vi "UDT_loggingModule_Postrun.vi"() -> (3 "Unit Test Framework Results":T1)   [LabVIEW 2017]
doc: "Use this template to create a user-defined test VI. Define your test requirements and wire the results to the <b>Result (Test)</b> control. Do not modify the <b>Unit Test Framework Results</b> indicator."
uses:
  <vilib>/utf/common/utf_test_result_troll.ctl
  <vilib>/utf/common/utf_test_result.ctl
  <vilib>/utf/common/utf_test_result_failure.ctl
  <vilib>/utf/common/utf_test_comparison_operators.ctl
  <vilib>/utf/common/utf_vi_tag.ctl
  RT/loggingModule/Queue/TypeDefs/queueFGVState.ctl
  RT/loggingModule/Queue/TypeDefs/message.ctl
  <vilib>/Control Software Solutions Ltd/UTF Helper/SubVIs/UTF Variant Equals.vi
  <vilib>/Control Software Solutions Ltd/UTF Helper/Unit Test Helper.lvlib
  RT/loggingModule/loggingModule.lvlib
  <vilib>/utf/NI_UnitTestFramework.lvlib
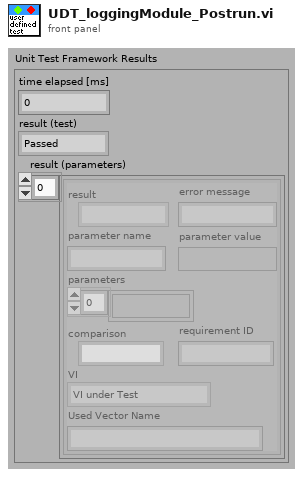
[diagram p1: front panel]
types:
  T1 = typedef "NI_UnitTestFramework.lvlib/utf_test_result_troll.ctl" = cluster{"time elapsed [ms]":u32, "result (test)":T2, "result (parameters)":T3[]}
  T2 = typedef "NI_UnitTestFramework.lvlib/utf_test_result.ctl" = enum16{"Passed", "Failed", "Error", "Skipped", "Not Processed"}
  T3 = typedef "NI_UnitTestFramework.lvlib/utf_test_result_failure.ctl" = cluster{"result":T2, "error message":string, "parameter name":string, "parameter value":variant, "parameters":variant[], "comparison":T4, "requirement ID":string, "VI":T5, "Used Vector Name":string}
  T4 = typedef "NI_UnitTestFramework.lvlib/utf_test_comparison_operators.ctl" = enum16{"=", "!=", ">", ">=", "<", "<=", "range", "symmetric tolerance", "asymmetric tolerance", "string contains", "string not contain", "array size", "string length", "array range", "by element", "array range (limit array)", "user-defined", "array contains", "array not contain", "vector length", "= (elm)", "!= (elm)", "= (case insensitive)", "!= (case insensitive)"}
  T5 = typedef "NI_UnitTestFramework.lvlib/utf_vi_tag.ctl" = enum16{"Setup VI", "VI under Test", "Teardown VI"}
  T6 = typedef "loggingModule.lvlib/message.ctl" = cluster{"calling module":string, "message":string, "data":variant}
  T7 = typedef "loggingModule.lvlib/queueFGVState.ctl" = enum16{"obtain", "enqueue low priority", "enqueue high priority", "dequeue", "release"}
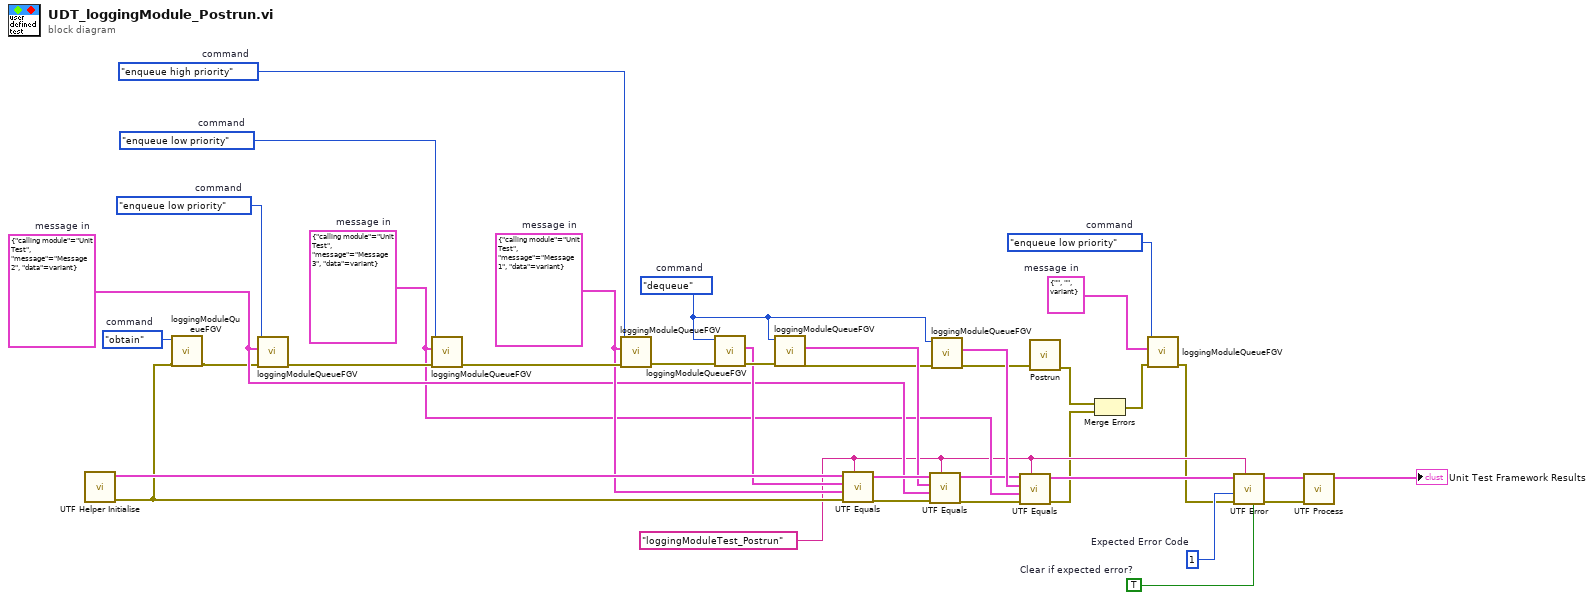
[diagram p0: block diagram]
diagram:
  w5 = TRUE  # Clear if expected error?
  w6 = 1  # Expected Error Code
  w11 = T6 {"calling module"="", "message"="", "data"=variant}  # message in
  w12 = queueFGVState."enqueue low priority"  # command
  w14 = queueFGVState."obtain"  # command
  w7 = "loggingModuleTest_Postrun"
  w22 = queueFGVState."dequeue"  # command
  w31 = T6 {"calling module"="Unit Test", "message"="Message 1", "data"=variant}  # message in
  w18 = T6 {"calling module"="Unit Test", "message"="Message 3", "data"=variant}  # message in
  w24 = T6 {"calling module"="Unit Test", "message"="Message 2", "data"=variant}  # message in
  w34 = queueFGVState."enqueue high priority"  # command
  w36 = queueFGVState."enqueue low priority"  # command
  w37 = queueFGVState."enqueue low priority"  # command
  n1 = call <vilib>:"UTF Helper Initialise.vi"() -> ("error out"=w16:errorcluster, "results array"=w32:T3[])  [unwired: 10 in]
  n2 = call "loggingModuleQueueFGV.vi"("error in (no error)"=w16, "command"=w14) -> ("error out"=w15:errorcluster)  [unwired: 8 in, 1 out]
  n3 = call "loggingModuleQueueFGV.vi"("error in (no error)"=w15, "message in"=w24, "command"=w37) -> ("error out"=w35:errorcluster)  [unwired: 7 in, 1 out]
  n4 = call "loggingModuleQueueFGV.vi"("error in (no error)"=w35, "message in"=w18, "command"=w36) -> ("error out"=w33:errorcluster)  [unwired: 7 in, 1 out]
  n5 = call "loggingModuleQueueFGV.vi"("error in (no error)"=w33, "message in"=w31, "command"=w34) -> ("error out"=w30:errorcluster)  [unwired: 7 in, 1 out]
  n6 = call "loggingModuleQueueFGV.vi"("error in (no error)"=w30, "command"=w22) -> ("error out"=w27:errorcluster, "message out"=w26:T6)  [unwired: 8 in]
  n7 = call "loggingModuleQueueFGV.vi"("error in (no error)"=w27, "command"=w22) -> ("error out"=w23:errorcluster, "message out"=w25:T6)  [unwired: 8 in]
  n8 = call-poly <vilib>:"UTF Equals.vi"("Parameter Name"=w7, "error in (no error)"=w16, "Test Value"=w31, "Input"=w26, "Input Results"=w32) -> ("error out"=w29:errorcluster, "Output Results"=w28:T3[])  [unwired: 5 in]
  n9 = call-poly <vilib>:"UTF Equals.vi"("Parameter Name"=w7, "error in (no error)"=w29, "Test Value"=w24, "Input"=w25, "Input Results"=w28) -> ("error out"=w19:errorcluster, "Output Results"=w20:T3[])  [unwired: 5 in]
  n10 = call "loggingModuleQueueFGV.vi"("error in (no error)"=w23, "command"=w22) -> ("error out"=w13:errorcluster, "message out"=w21:T6)  [unwired: 8 in]
  n11 = call-poly <vilib>:"UTF Equals.vi"("Parameter Name"=w7, "error in (no error)"=w19, "Test Value"=w18, "Input"=w21, "Input Results"=w20) -> ("error out"=w3:errorcluster, "Output Results"=w9:T3[])  [unwired: 5 in]
  n12 = call "Postrun.vi"("error in (no error)"=w13) -> ("error out"=w4:errorcluster)  [unwired: 10 in]
  n13 = Merge Errors(w4, w3) -> (w2:errorcluster)
  n14 = call "loggingModuleQueueFGV.vi"("error in (no error)"=w2, "message in"=w11, "command"=w12) -> ("error out"=w1:errorcluster)  [unwired: 7 in, 1 out]
  n15 = call <vilib>:"UTF Error.vi"("Clear if expected error?"=w5, "Parameter Name"=w7, "error in (no error)"=w1, "Expected Error Code"=w6, "Input Results"=w9) -> ("error out"=w10:errorcluster, "Output Results"=w8:T3[])  [unwired: 5 in]
  n16 = call <vilib>:"UTF Process.vi"("error in (no error)"=w10, "results array"=w8) -> ("Unit Test Framework Results"=→"Unit Test Framework Results":T1)  [unwired: 9 in]
